vi "SSL Detection Frame Simple Estimator Cameras Number.vi"(7 "id":u32, 9 "camera_id":u32, 10 "Detection Frame In":T1, 11 "Enable":bool) -> (3 "Detection Frame Out":T1)   [LabVIEW 2016]
uses:
  SSL Detection Frame.ctl
  SSL Detection Robot.ctl
  SSL Detection Ball.ctl
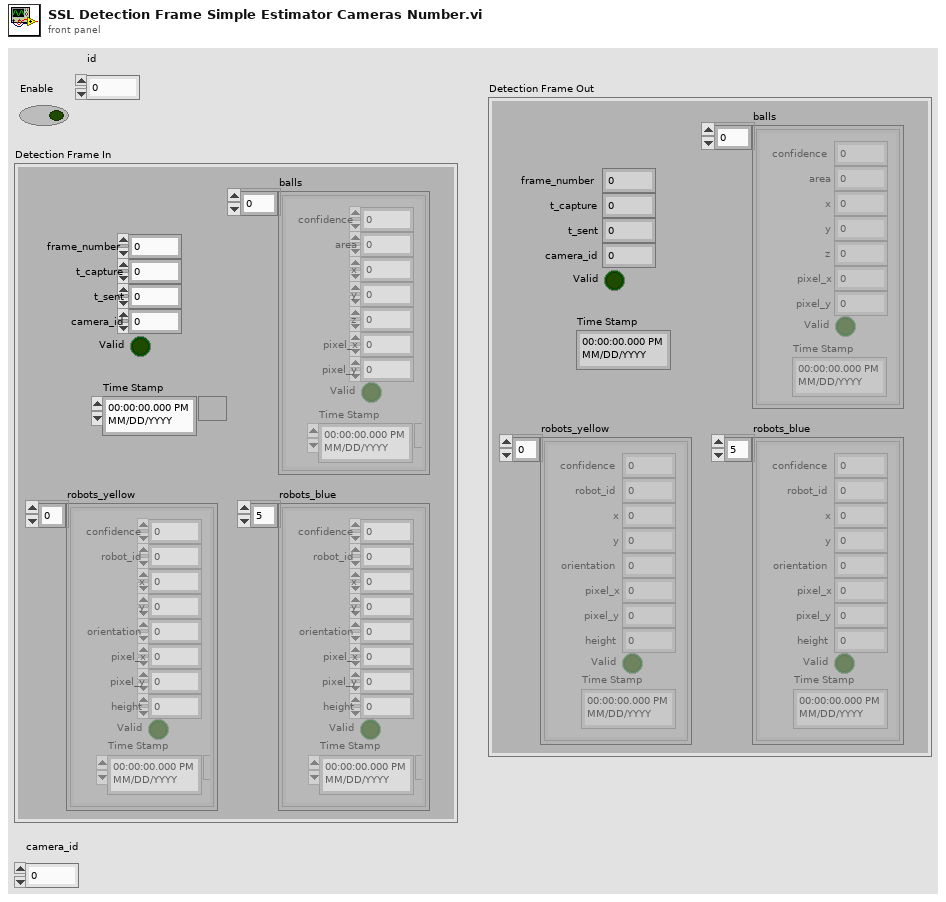
[diagram p1: front panel]
types:
  T1 = typedef "SSL Detection Frame.ctl" = cluster{"frame_number":u32, "t_capture":dbl, "t_sent":dbl, "camera_id":u32, "robots_yellow":T2[], "robots_blue":T2[], "balls":T3[], "Valid":bool, "Time Stamp":timestamp}
  T2 = typedef "SSL Detection Robot.ctl" = cluster{"x":dbl, "robot_id":u32, "confidence":sgl, "y":sgl, "orientation":sgl, "pixel_x":sgl, "pixel_y":sgl, "height":sgl, "Valid":bool, "Time Stamp":timestamp}
  T3 = typedef "SSL Detection Ball.ctl" = cluster{"x":sgl, "area":u32, "confidence":sgl, "y":sgl, "z":sgl, "pixel_x":sgl, "pixel_y":sgl, "Valid":bool, "Time Stamp":timestamp}
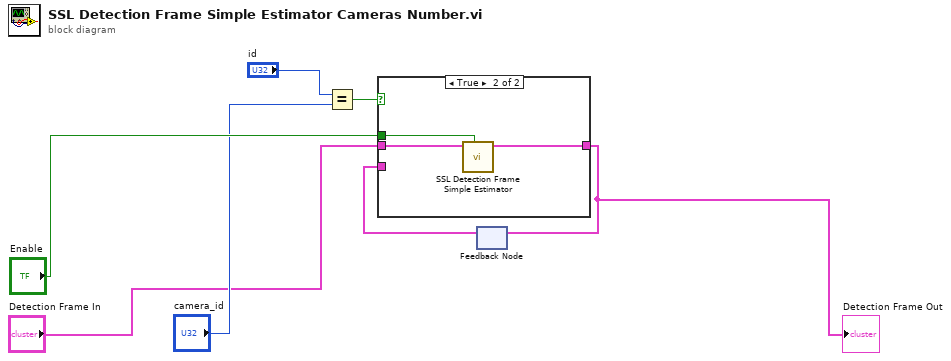
[diagram p0: block diagram]
diagram:
  n1 = Equal?(x="id", y="camera_id") -> (x = y?=w3:bool)
  n2 = feedback #1() -> (w1:T1)  [unwired: 1 in]
  n3 = case shown="True" w3 {
    tunnel: "Detection Frame In" -> [_ w11]
    tunnel: [w8 w10] -> w7
    tunnel: w1 -> [w8 _]
    tunnel: "Enable" -> [_ w9]
    frame False {
    }
    frame True {
      n4 = call "SSL Detection Frame Simple Estimator.vi"("Enable"=w9, "Detection Frame In"=w11) -> ("Detection Frame Out"=w10:T1)  [unwired: 8 in, 1 out]
    }
  }
  "Detection Frame Out" <- w7
  n5 = feedback-in #1(w7) -> ()
